vi "ShortestPath.vi"() -> ()   [LabVIEW 2014]
uses:
  <userlib>/AdvancedDataStructures/ClassBased/Applications/Occupancy/OccupancyMap/OccupancyMap.lvclass
  <userlib>/AdvancedDataStructures/ClassBased/Applications/Occupancy/OccupancyMap/parameters.ctl
  <userlib>/AdvancedDataStructures/ClassBased/Applications/Occupancy/Rectangle/Rectangle.lvclass
  <userlib>/AdvancedDataStructures/ClassBased/Graph/Graph.lvclass
panel:
  in  "Solve":bool
  out "Occupancy Map":picture
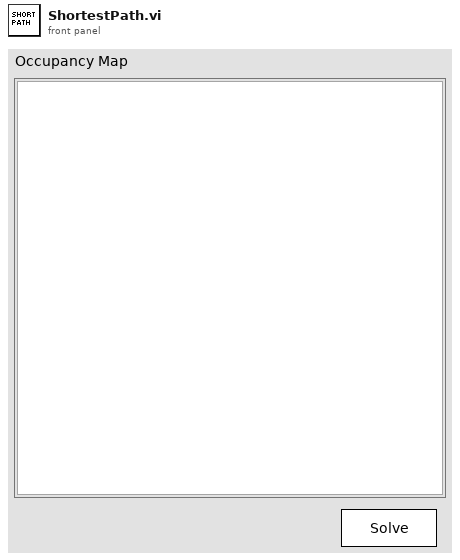
[diagram p1: front panel]
types:
  T1 = cluster{"left":i16, "top":i16, "right":i16, "bottom":i16}
  T2 = cluster{"Left":dbl, "Right":dbl, "Top":dbl, "Bottom":dbl}
  T3 = cluster{"Width":i16, "Style":enum32{"Solid", "Dash", "Dot", "DashDot", "DashDotDot"}}
  T4 = typedef "OccupancyMap.lvclass/parameters.ctl" = cluster{"MapResolution":cluster{"resX":dbl, "resY":dbl}, "StartLocation":cluster{"X":dbl, "Y":dbl}, "Goal":cluster{"X":dbl, "Y":dbl}, "MapBoundaries":cluster{"Left":dbl, "Right":dbl, "Top":dbl, "Bottom":dbl}}
  T5 = cluster{"Width":u16, "Style":enum32{"Solid", "Dash", "Dot", "DashDot", "DashDotDot"}}
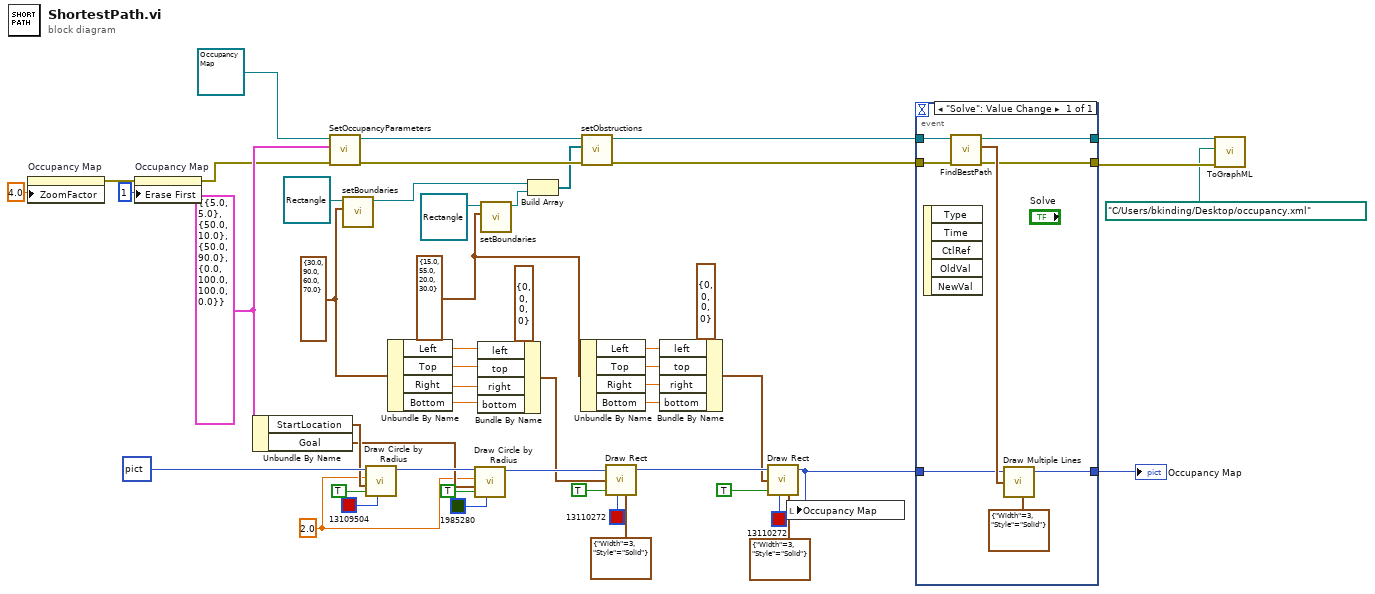
[diagram p0: block diagram]
diagram:
  w10 = T2 {"Left"=15.0, "Right"=55.0, "Top"=20.0, "Bottom"=30.0} ("Boundaries")
  w15 = T2 {"Left"=30.0, "Right"=90.0, "Top"=60.0, "Bottom"=70.0} ("Boundaries")
  w42 = sgl 2.0 ("Zoom Factor")
  w49 = T4 {"MapResolution"={"resX"=5.0, "resY"=5.0}, "StartLocation"={"X"=50.0, "Y"=10.0}, "Goal"={"X"=50.0, "Y"=90.0}, "MapBoundaries"={"Left"=0.0, "Right"=100.0, "Top"=100.0, "Bottom"=0.0}} ("Parameters")
  n1 = property on="Occupancy Map" class="Pict"("ZoomFactor"=sgl 4.0 ("Zoom Factor")) -> (error out=w30:errorcluster)  [unwired: 2 in, 1 out]
  n2 = property on="Occupancy Map" class="Pict"(error in=w30, "Erase First"=u8 1) -> (error out=w29:errorcluster)  [unwired: 1 in, 1 out]
  n3 = Unbundle By Name(w49) -> ("StartLocation"=w48:cluster{"X":dbl, "Y":dbl}, "Goal"=w46:cluster{"X":dbl, "Y":dbl})
  n4 = call <userlib>:"SetOccupancyParameters.vi"("error in (no error)"=w29, "Parameters"=w49, "OccupancyMap in"=refnum<class "OccupancyMap.lvclass"> refnum) -> ("error out"=w38:errorcluster, "OccupancyMap out"=w39:refnum<class "OccupancyMap.lvclass">)  [unwired: 7 in]
  n5 = call <userlib>:"setBoundaries.vi"("Boundaries"=w15, "Rectangle in"=refnum<class "Rectangle.lvclass"> refnum ("Rectangle.lvclass")) -> ("Rectangle out"=w35:refnum<class "Rectangle.lvclass">)  [unwired: 8 in, 1 out]
  n6 = call <vilib>:"Draw Circle by Radius.vi"("color(black)"=u32 13109504, "fill?(F)"=TRUE, "pixel center"=w48, "radius"=w42, "picture"=picture data[5B] ("2D Picture")) -> ("new picture"=w47:picture)  [unwired: 6 in]
  n7 = Unbundle By Name(w15) -> ("Left"=w34:dbl, "Top"=w33:dbl, "Right"=w32:dbl, "Bottom"=w31:dbl)
  n8 = call <vilib>:"Draw Circle by Radius.vi"("color(black)"=u32 1985280, "fill?(F)"=TRUE, "pixel center"=w46, "radius"=w42, "picture"=w47) -> ("new picture"=w25:picture)  [unwired: 6 in]
  n9 = Bundle By Name(cluster=T1 {"left"=0, "top"=0, "right"=0, "bottom"=0} ("rect"), "left"=w34, "top"=w33, "right"=w32, "bottom"=w31) -> (w17:T1)
  n10 = call <userlib>:"setBoundaries.vi"("Boundaries"=w10, "Rectangle in"=refnum<class "Rectangle.lvclass"> refnum ("Rectangle.lvclass")) -> ("Rectangle out"=w13:refnum<class "Rectangle.lvclass">)  [unwired: 8 in, 1 out]
  n11 = Build Array(w35, w13) -> (w37:refnum<class "Rectangle.lvclass">[])
  n12 = Unbundle By Name(w10) -> ("Left"=w11:dbl, "Top"=w9:dbl, "Right"=w8:dbl, "Bottom"=w7:dbl)
  n13 = call <userlib>:"setObstructions.vi"("error in (no error)"=w38, "Obstructions"=w37, "OccupancyMap in"=w39) -> ("error out"=w41:errorcluster, "OccupancyMap out"=w40:refnum<class "OccupancyMap.lvclass">)  [unwired: 7 in]
  n14 = call <vilib>:"Draw Rect.vi"("picture"=w25, "rect"=w17, "fill?(F)"=TRUE, "color(black)"=u32 13110272, "pen"=T3 {"Width"=3, "Style"=enum."Solid"}) -> ("new picture"=w23:picture)  [unwired: 4 in]
  n15 = Bundle By Name(cluster=T1 {"left"=0, "top"=0, "right"=0, "bottom"=0} ("rect"), "left"=w11, "top"=w9, "right"=w8, "bottom"=w7) -> (w6:T1)
  n16 = call <vilib>:"Draw Rect.vi"("picture"=w23, "rect"=w6, "fill?(F)"=TRUE, "color(black)"=u32 13110272, "pen"=T3 {"Width"=3, "Style"=enum."Solid"}) -> ("new picture"=w19:picture)  [unwired: 4 in]
  n17 = local write "Occupancy Map"(w19) -> ()
  n18 = event shown="[0] \"Solve\": Value Change" {
    selector: _ -> [_]
    dyn-events: _ -> [_]
    timeout: _ -> [_]
    tunnel: w41 -> [w58]
    tunnel: w40 -> [w57]
    tunnel: [w55] -> w20
    tunnel: w19 -> [w54]
    tunnel: [w53] -> w3
    tunnel: [w52] -> w2
    event "Solve": Value Change {
      n19 = event-data() -> ()  [unwired: 1 in, 5 out]
      n20 = call <userlib>:"FindBestPath.vi"("error in (no error)"=w58, "OccupancyMap in"=w57) -> ("error out"=w52:errorcluster, "path"=w59:cluster{"X":dbl, "Y":dbl}[], "OccupancyMap out"=w53:refnum<class "OccupancyMap.lvclass">)  [unwired: 6 in, 1 out]
      n21 = call <vilib>:"Draw Multiple Lines.vi"("picture"=w54, "line endpoints"=w59, "pen"=T5 {"Width"=3, "Style"=enum."Solid"}) -> ("new picture"=w55:picture)  [unwired: 6 in]
    }
  }
  "Occupancy Map" <- w20
  n22 = call <userlib>:"ToGraphML.vi"("error in (no error)"=w2, "file"=path "C:/Users/bkinding/Desktop/occupancy.xml", "Graph in"=w3) -> ()  [unwired: 7 in, 2 out]
